vi "Button Refs.vi"(8 "error in":errorcluster, 10 "Disabled":T1(ring), 11 "ATM Data":T2={"UI Refs"={"Right Buttons"=refnum, "Left Buttons"=refnum, "User Input"=refnum, "ATM Messages"=refnum, "Left Menu"=refnum, "Right Menu"=refnum, "Enter"=refnum}, "Map"={}, "Login Valid?"=FALSE, "Queue Message"=refnum, "State"=enum."None", "User"={"Pin"="", "First Name"="", "Last Name"="", "Balance"=0.0, "Login Valid?"=FALSE}, "Main States"={"Message"="Initialize", "Data"=variant}}) -> (0 "error out":errorcluster, 3 "ATM Data Out":T2={"UI Refs"={"Right Buttons"=refnum, "Left Buttons"=refnum, "User Input"=refnum, "ATM Messages"=refnum, "Left Menu"=refnum, "Right Menu"=refnum, "Enter"=refnum}, "Map"={}, "Login Valid?"=FALSE, "Queue Message"=refnum, "State"=enum."None", "User"={"Pin"="", "First Name"="", "Last Name"="", "Balance"=0.0, "Login Valid?"=FALSE}, "Main States"={"Message"="Initialize", "Data"=variant}})   [LabVIEW 2020, in "ATM Machine.lvlib"]
uses:
  ATM Machine.lvlib
  Cluster - ATM Machine Data.ctl
  Users/khemr/OneDrive/Desktop/Labview Training/CLD/New ATM_KR/ATM Machine/Cluster - Message Cluster.ctl
  Enum - ATM States.ctl
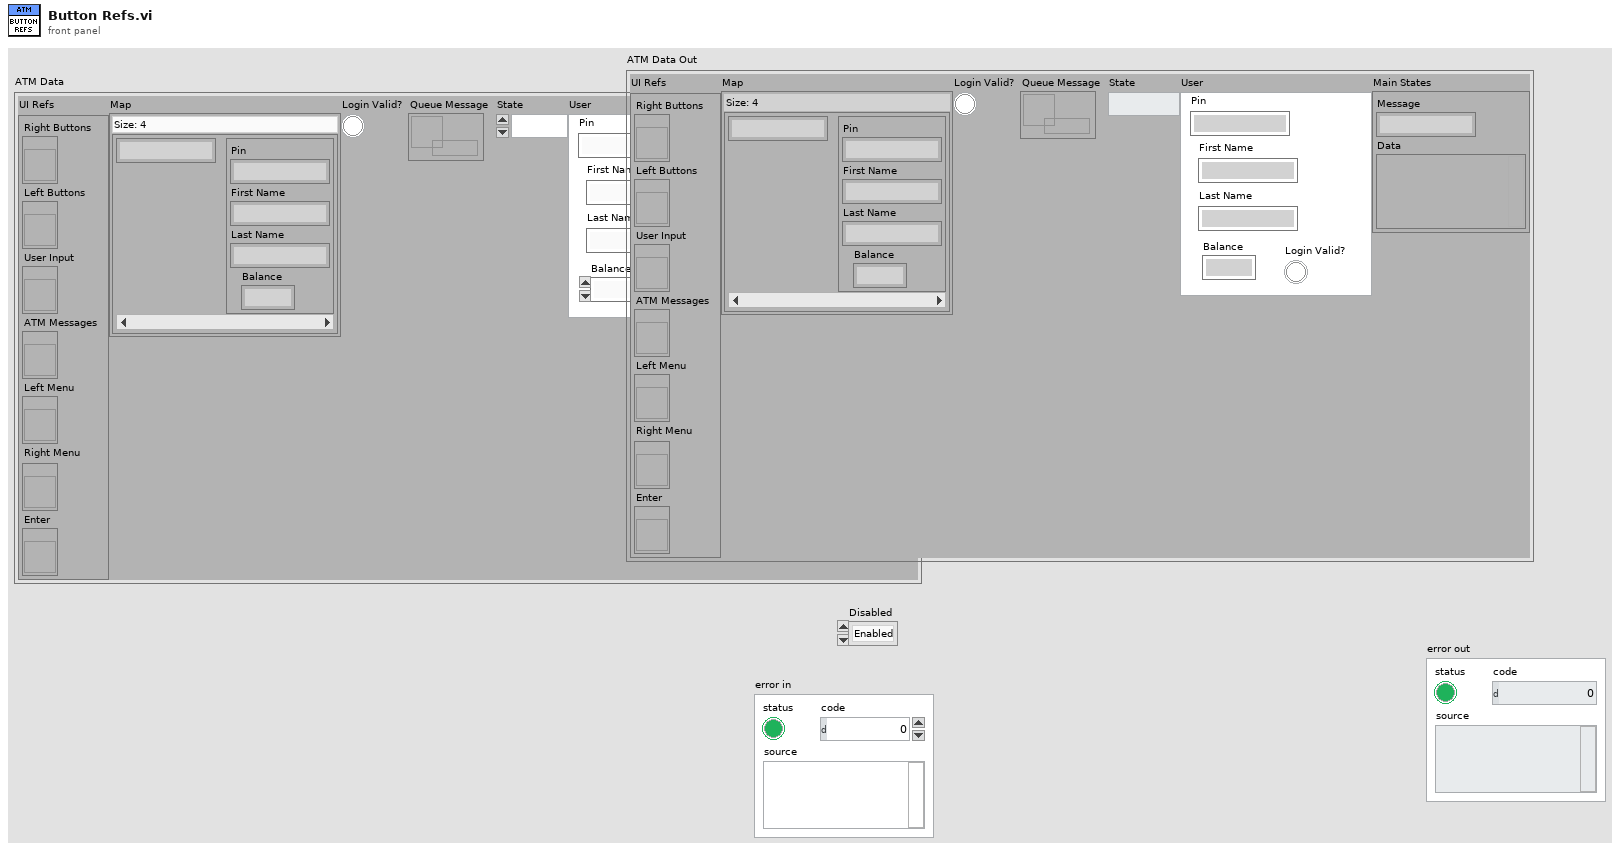
[diagram p1: front panel]
types:
  T1 = enum8{"Enabled", "Disabled", "Disabled and Grayed Out"}
  T2 = typedef "ATM Machine.lvlib/Cluster - ATM Machine Data.ctl" = cluster{"UI Refs":cluster{"Right Buttons":refnum<vi>, "Left Buttons":refnum<vi>, "User Input":refnum<vi>, "ATM Messages":refnum<vi>, "Left Menu":refnum<vi>, "Right Menu":refnum<vi>, "Enter":refnum<vi>}, "Map":map{string, cluster{"Pin":string, "First Name":string, "Last Name":string, "Balance":dbl}}, "Login Valid?":bool, "Queue Message":refnum<queue>, "State":T3, "User":cluster{"Pin":string, "First Name":string, "Last Name":string, "Balance":dbl, "Login Valid?":bool}, "Main States":cluster{"Message":string, "Data":variant}}
  T3 = typedef "ATM Machine.lvlib/Enum - ATM States.ctl" = enum16{"None", "Deposit", "Withdraw", "Card Inserted", "Balance Inquiry", "Return Card and Terminate", "Fast Cash"}
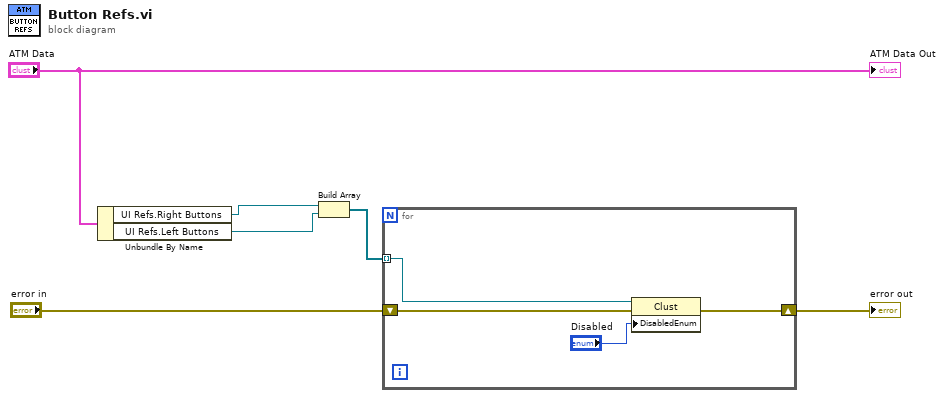
[diagram p0: block diagram]
diagram:
  n1 = Unbundle By Name("ATM Data") -> ("UI Refs.Right Buttons"=w2:refnum<vi>, "UI Refs.Left Buttons"=w1:refnum<vi>)
  n2 = Build Array(w2, w1) -> (w3:refnum<vi>[])
  n3 = for {
    shift-right: [w9] -> w5
    shift-left: "error in" -> [w10]
    tunnel: w3 -> [w8] mode=indexing
    n4 = property class="Clust"(reference=w8, error in=w10, "DisabledEnum"="Disabled") -> (error out=w9:errorcluster)  [unwired: 1 out]
  }
  "error out" <- w5
  "ATM Data Out" <- "ATM Data"
